vi "1_RGT_Text.vi"() -> ()   [LabVIEW 2014]
uses:
  <vilib>/Utility/NIReport.llb/NI_report.lvclass
  <vilib>/Utility/NIReport.llb/Append Report Text (str wrap).vi
panel:
  in  "font settings":T1={"Charset (-1)"=-1, "Weight (-1)"=-1, "Name"="Arial", "Size"="30 "}
  in  "text options":T2={"Italic"=enum."Italic Unchanged", "Strike Through"=enum."Strike Through Unchanged", "Underline"=enum."Underline Unchanged", "Bold"=enum."Bold On"}
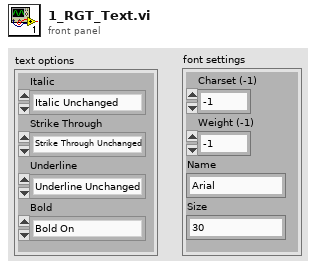
[diagram p1: front panel]
types:
  T1 = cluster{"Charset (-1)":i16, "Weight (-1)":i16, "Name":string, "Size":string}
  T2 = cluster{"Italic":enum16{"Italic Unchanged", "Italic On", "Italic Off"}, "Strike Through":enum16{"Strike Through Unchanged", "Strike Through On", "Strike Through Off"}, "Underline":enum16{"Underline Unchanged", "Underline On", "Underline Off"}, "Bold":enum16{"Bold Unchanged", "Bold On", "Bold Off"}}
  T3 = enum16{"Standard Report", "HTML", "Word", "Excel"}
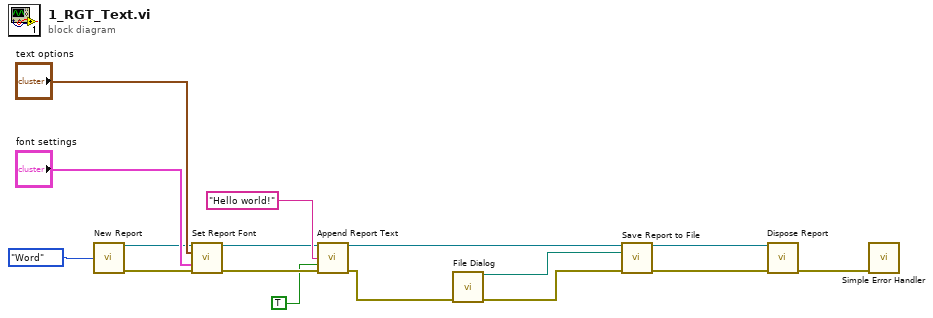
[diagram p0: block diagram]
diagram:
  n1 = call <vilib>:"New Report.vi"("report type"=T3."Word") -> ("report out"=w11:refnum<class "NI_report.lvclass">, "error out"=w16:errorcluster)  [unwired: 13 in]
  n2 = call-dynamic "Set Report Font.vi"("report in"=w11, "text options"="text options", "font settings"="font settings", "error in (no error)"=w16) -> ("report out"=w10:refnum<class "NI_report.lvclass">, "error out"=w15:errorcluster)  [unwired: 9 in, 1 out]
  n3 = call-poly <vilib>:"Append Report Text.vi"("report in"=w10, "text"="Hello world!", "append on new line? (F)"=TRUE, "error in (no error)"=w15) -> ("report out"=w4:refnum<class "NI_report.lvclass">, "error out"=w2:errorcluster)  [unwired: 8 in, 2 out]
  n4 = call "File Dialog"("error in"=w2) -> ("selected path"=w3:path, "error out"=w1:errorcluster)  [unwired: 11 in, 2 out]
  n5 = call-dynamic "Save Report to File.vi"("report in"=w4, "report file path"=w3, "error in (no error)"=w1) -> ("report out"=w6:refnum<class "NI_report.lvclass">, "error out"=w5:errorcluster)  [unwired: 11 in]
  n6 = call-dynamic "Dispose Report.vi"("report in"=w6, "error in (no error)"=w5) -> ("error out"=w8:errorcluster)  [unwired: 13 in]
  n7 = call <vilib>:"Simple Error Handler.vi"("error in (no error)"=w8) -> ()  [unwired: 4 in, 5 out]
